vi "CRYGroup Manipulate.vi"(6 "sData In":string[](array[string]), 7 "sAction":string, 8 "sOption":string, 9 "nData":i32[](array[numeric]), 10 "Type":enum16{"Curves", "Values", "Results", "WFM"}(ring), 11 "Tree in":refnum<vi>) -> (0 "bData out":bool, 1 "sData Out":string[](array[string]), 2 "nData Out":i32[](array[numeric]), 3 "Tree Out":refnum<vi>)   [LabVIEW 2013]
uses:
  Global/CRYCurve Library Global.vi
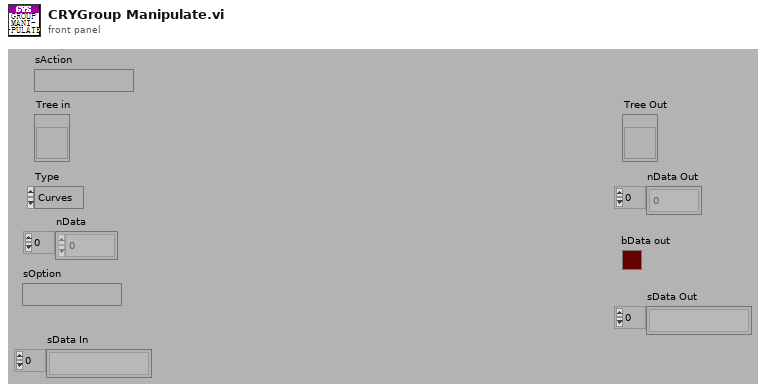
[diagram p1: front panel]
types:
  T1 = enum16{"OK", "Yes", "YesNo", "YesNoCancel", "ReplaceAppend"}
  T2 = typedef "CRYCurveLib Info Cluster.ctl" = cluster{"GroupingState":string}
  T3 = typedef "CRYStep.ctl" = cluster{"No.VI":i32, "Category":string, "StepName":string, "Seq setup flattened":string, "Comment":string, "Steps config.":bool[], "Jump config":i32[], "Start":dbl, "Increment":dbl, "Name":string, "Unit":string, "Y data":u16, "Y prefix":string, "Y dB ref":dbl, "Y unit":string, "Repeat State Array":cluster{"Start":dbl, "Increment":dbl, "Count":i32, "Num":i32}[]}
  T4 = cluster{"Tags":string[], "StepNo&Category":string}[]
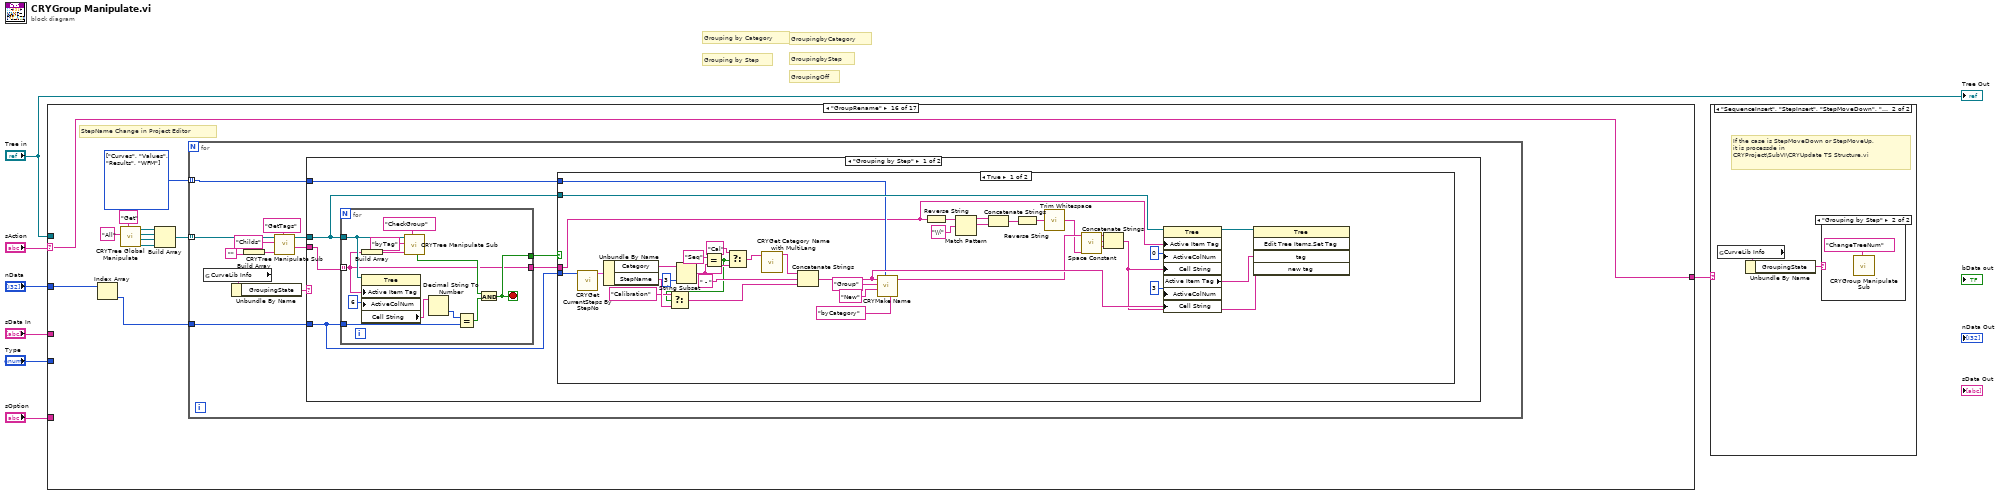
[diagram p0: block diagram]
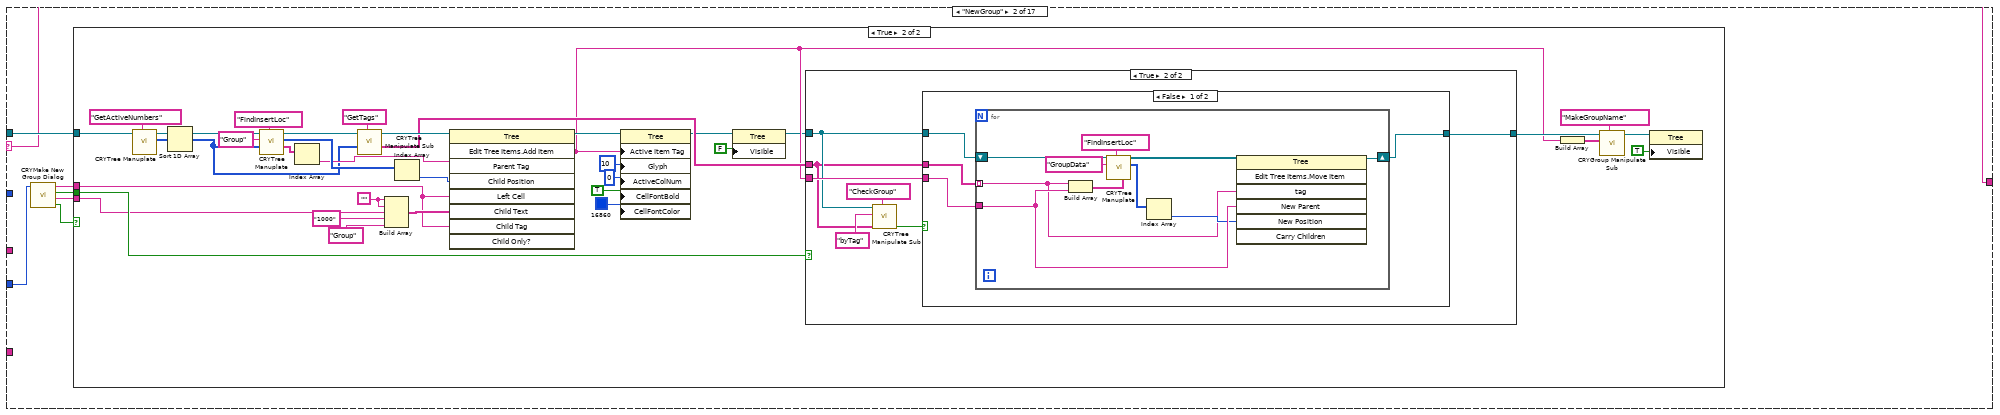
[diagram p5: hidden frame]
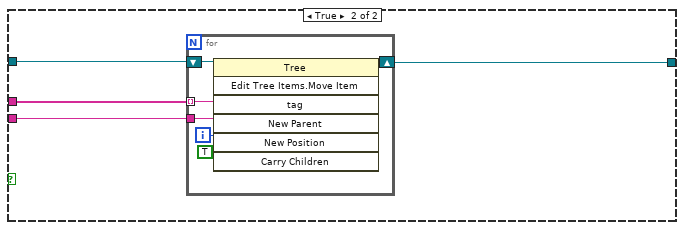
[diagram p8: hidden frame]
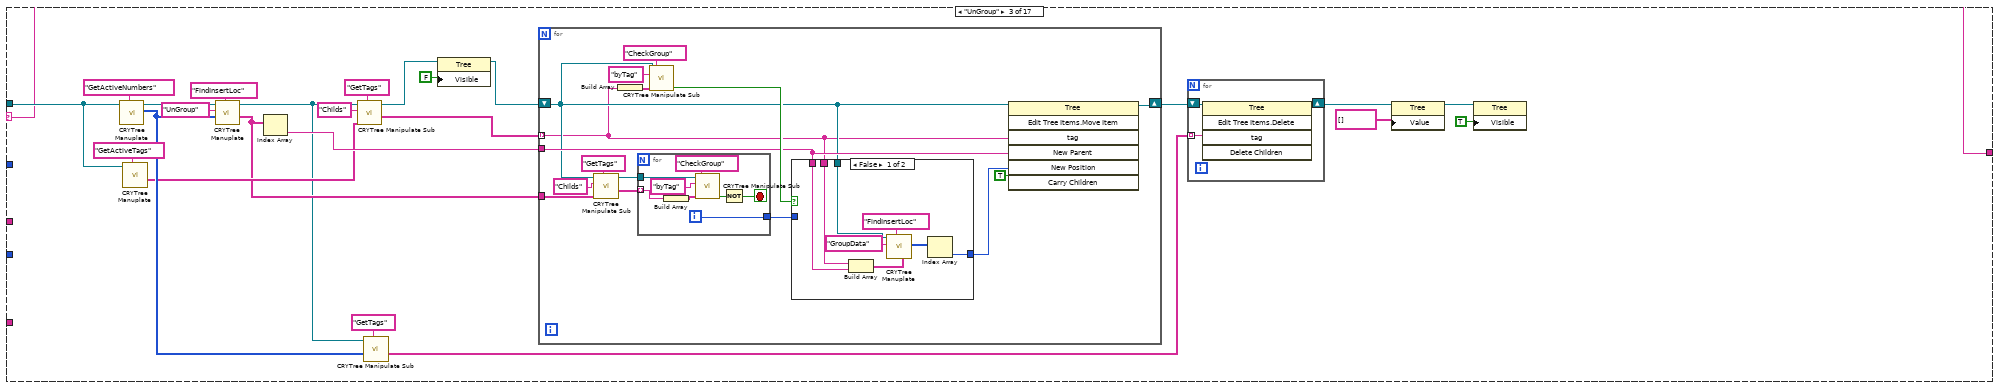
[diagram p9: hidden frame]
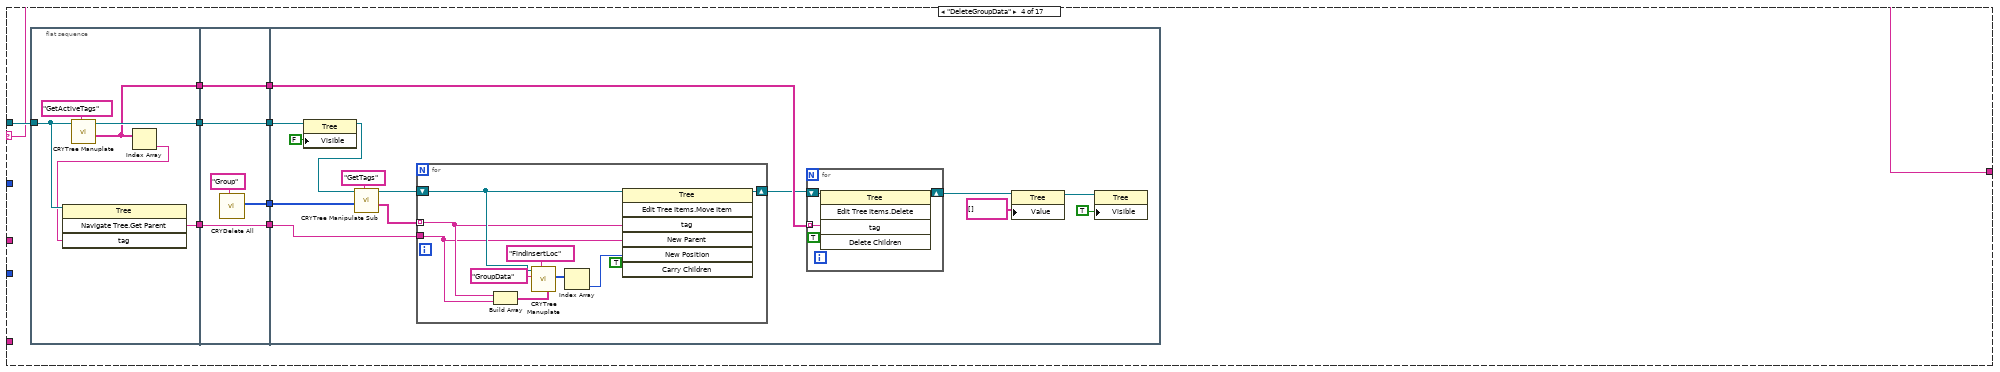
[diagram p11: hidden frame]
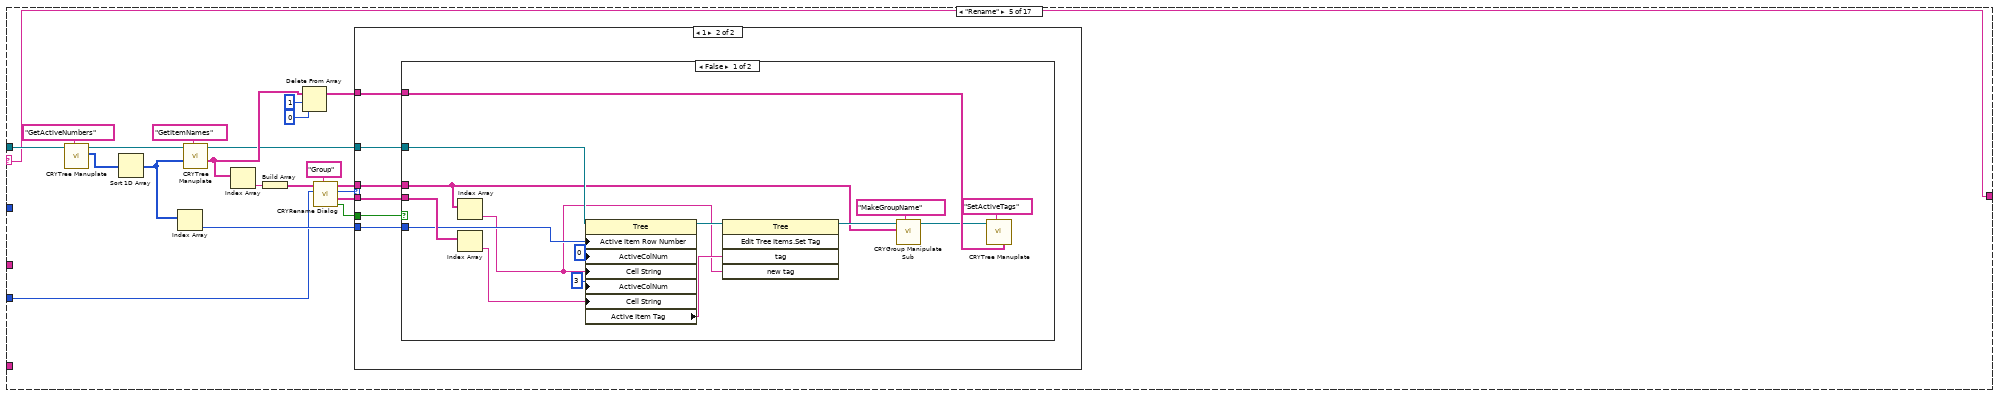
[diagram p12: hidden frame]
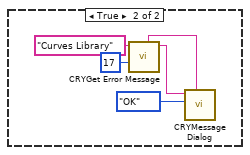
[diagram p14: hidden frame]
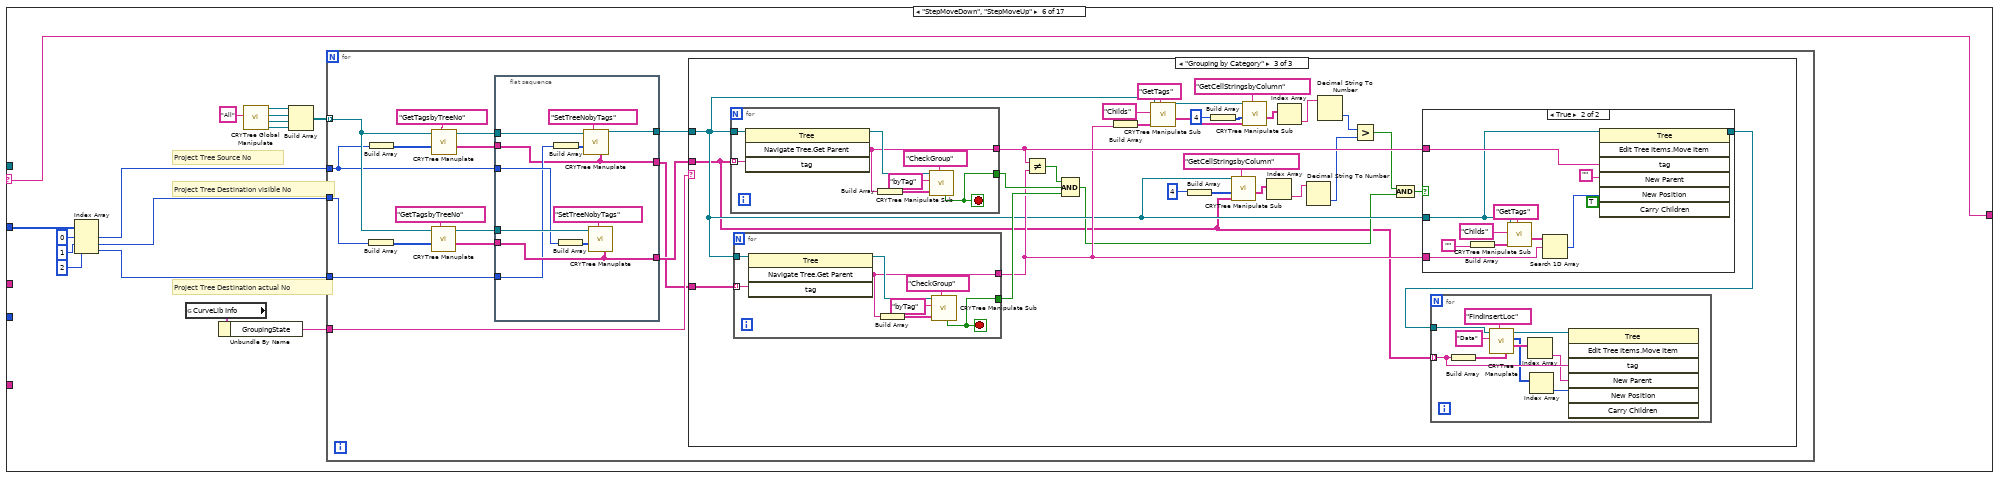
[diagram p15: hidden frame]
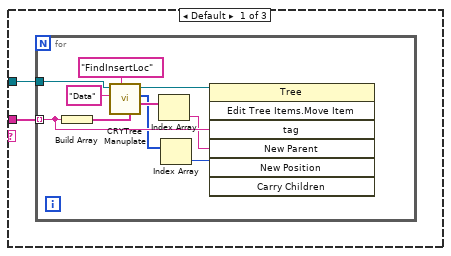
[diagram p16: hidden frame]
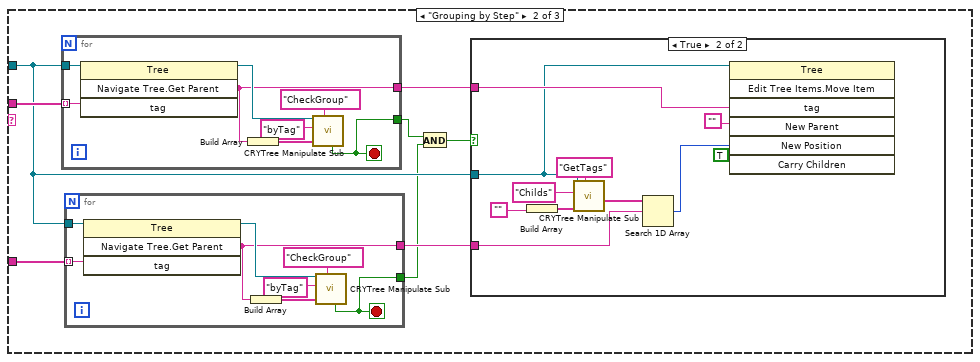
[diagram p17: hidden frame]
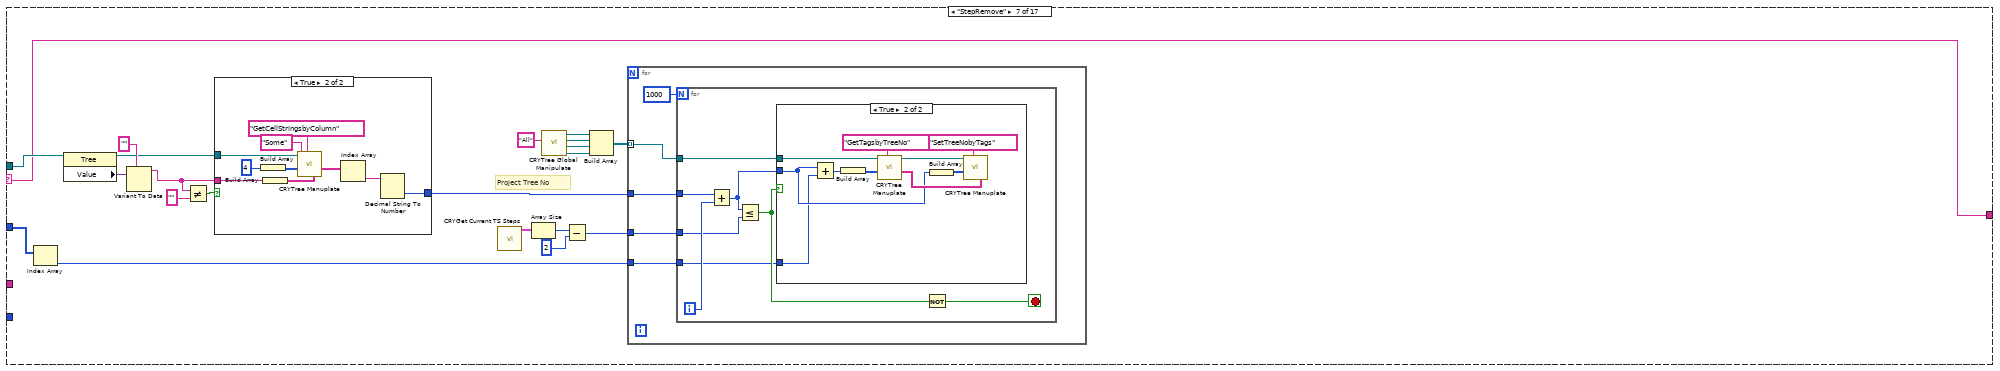
[diagram p20: hidden frame]
diagram:
  # "Grouping by Step"
  # "Grouping by Category"
  # "GroupingOff"
  # "GroupingbyStep"
  # "GroupingbyCategory"
  n1 = case shown="\"GroupRename\"" "sAction" {
    selector: "sAction" -> [w8 w9 w84 w145 w193 w242 w398 w452 w501 w555 w568 w581 w601 w709 w776 w835 w902]
    tunnel: "nData" -> [_ _ _ _ _ w247 w400 _ w503 w564 w569 w584 _ _ w790 w837 w916]
    tunnel: "Tree in" -> [_ w12 w88 w146 w202 _ w407 w459 w510 w562 w570 w585 _ _ w791 _ w937]
    tunnel: "Type" -> [_ w10 _ _ w194 _ _ _ _ _ _ _ _ _ _ _ w909]
    tunnel: "sOption" -> [_ _ _ _ _ _ _ _ _ _ _ _ _ w710 _ _ _]
    tunnel: [w8 w9 w84 w145 w193 w242 w398 w452 w501 w555 w568 w581 w601 w709 w776 w835 w902] -> w2
    tunnel: "sData In" -> [_ _ _ _ _ _ _ _ _ _ _ _ _ _ _ _ _]
    frame "None", Default {
    }
    frame "NewGroup" {
      n2 = call "CRYMake New Group Dialog.vi"("Type"=w10) -> ("Return Flag"=w14:bool, "Org Group Name"=w11:string, "InGroup?"=w13:bool, "New Group Name"=w15:string)  [unwired: 7 in]
      n3 = case shown="True" w14 {
        tunnel: w12 -> [_ w20]
        tunnel: w15 -> [_ w36]
        tunnel: w13 -> [_ w45]
        tunnel: w11 -> [_ w29]
        frame False {
        }
        frame True {
          w30 = ""
          n4 = call "CRYTree Manuplate.vi"("sAction"="GetActiveNumbers", "Tree in"=w20) -> ("nData Out"=w31:i32[], "Tree Out"=w46:refnum<vi>)  [unwired: 6 in, 2 out]
          n5 = Sort 1D Array(array=w31) -> (sorted array=w23:i32[])
          n6 = call "CRYTree Manuplate.vi"("sAction"="FindInsertLoc", "nData"=w23, "sOption"="Group" ("sData"), "Tree in"=w46) -> ("sData Out"=w39:string[], "nData Out"=w41:i32[], "Tree Out"=w37:refnum<vi>)  [unwired: 4 in, 1 out]
          n7 = Index Array(array=w39) -> (element=w35:string)  [unwired: 1 in]
          n8 = call "CRYTree Manipulate Sub.vi"("sAction"="GetTags", "nData"=w23, "Tree in"=w37) -> ("sData Out"=w42:string[], "Tree Out"=w43:refnum<vi>)  [unwired: 4 in, 3 out]
          n9 = Build Array(w30, w30, w29, "1000" ("element"), "Group" ("element")) -> (w49:string[])
          n10 = Index Array(array=w41) -> (element=w40:i32)  [unwired: 1 in]
          n11 = invoke class="Tree" method="Edit Tree Items.Add Item"(reference=w43, "Parent Tag"=w35, "Child Position"=w40, "Left Cell"=w36, "Child Text"=w49, "Child Tag"=w36) -> (reference out=w51:refnum<vi>, "Edit Tree Items:Add Item"=w26:string)  [unwired: 3 in, 7 out]
          n12 = property class="Tree"(reference=w51, "Active Item Tag"=w26, "Glyph"=10 ("Active Item:Symbol Index"), "ActiveColNum"=0 ("Active Cell:Active Column Number"), "CellFontBold"=TRUE ("Active Cell:Cell Font:Bold"), "CellFontColor"=u32 16860) -> (reference out=w18:refnum<vi>)  [unwired: 1 in, 1 out]
          n13 = property class="Tree"(reference=w18, "Visible"=FALSE) -> (reference out=w17:refnum<vi>)  [unwired: 1 in, 1 out]
          n14 = case shown="True" w45 {
            tunnel: w26 -> [_ w59]
            tunnel: w17 -> [w52 w55]
            tunnel: w42 -> [_ w54]
            tunnel: [w52 w58] -> w27
            frame False {
            }
            frame True {
              n15 = call "CRYTree Manipulate Sub.vi"("sAction"="CheckGroup", "sData"=w54, "sOption"="byTag", "Tree in"=w55) -> ("bData out"=w53:bool)  [unwired: 3 in, 4 out]
              n16 = case shown="False" w53 {
                tunnel: w59 -> [w61 w77]
                tunnel: [w60 w76] -> w58
                tunnel: w55 -> [w63 w75]
                tunnel: w54 -> [w62 w74]
                frame False {
                  n17 = for {
                    tunnel: w62 -> [w69] mode=indexing
                    tunnel: w61 -> [w72]
                    shift-right: [w71] -> w60
                    shift-left: w63 -> [w68]
                    n18 = Build Array(w69, w72) -> (w65:string[])
                    n19 = call "CRYTree Manuplate.vi"("sData"=w65, "sAction"="FindInsertLoc", "sOption"="GroupData", "Tree in"=w68) -> ("nData Out"=w64:i32[], "Tree Out"=w73:refnum<vi>)  [unwired: 4 in, 2 out]
                    n20 = Index Array(array=w64) -> (element=w70:i32)  [unwired: 1 in]
                    n21 = invoke class="Tree" method="Edit Tree Items.Move Item"(reference=w73, "tag"=w69, "New Parent"=w72, "New Position"=w70) -> (reference out=w71:refnum<vi>)  [unwired: 3 in, 6 out]
                  }
                }
                frame True {
                  n22 = for {
                    tunnel: w77 -> [w81]
                    tunnel: w74 -> [w82] mode=indexing
                    shift-right: [w78] -> w76
                    shift-left: w75 -> [w83]
                    i -> [w80]
                    n23 = invoke class="Tree" method="Edit Tree Items.Move Item"(reference=w83, "tag"=w82, "New Parent"=w81, "New Position"=w80, "Carry Children"=TRUE ("Carry Children?")) -> (reference out=w78:refnum<vi>)  [unwired: 2 in, 6 out]
                  }
                }
              }
            }
          }
          n24 = Build Array(w26) -> (w16:string[])
          n25 = call "CRYGroup Manipulate Sub.vi"("sAction"="MakeGroupName", "sData"=w16, "Tree in"=w27) -> ("Tree Out"=w21:refnum<vi>)  [unwired: 4 in, 4 out]
          n26 = property class="Tree"(reference=w21, "Visible"=TRUE) -> ()  [unwired: 1 in, 2 out]
        }
      }
    }
    frame "UnGroup" {
      n27 = call "CRYTree Manuplate.vi"("sAction"="GetActiveNumbers", "Tree in"=w88) -> ("nData Out"=w98:i32[], "Tree Out"=w106:refnum<vi>)  [unwired: 6 in, 2 out]
      n28 = call "CRYTree Manuplate.vi"("sAction"="GetActiveTags", "Tree in"=w88) -> ("sData Out"=w96:string[])  [unwired: 6 in, 3 out]
      n29 = call "CRYTree Manuplate.vi"("sAction"="FindInsertLoc", "nData"=w98, "sOption"="UnGroup" ("sData"), "Tree in"=w106) -> ("sData Out"=w95:string[], "Tree Out"=w92:refnum<vi>)  [unwired: 4 in, 2 out]
      n30 = Index Array(array=w95) -> (element=w102:string)  [unwired: 1 in]
      n31 = call "CRYTree Manipulate Sub.vi"("sAction"="GetTags", "sData"=w96, "sOption"="Childs" ("sData"), "Tree in"=w92) -> ("sData Out"=w103:string[], "Tree Out"=w86:refnum<vi>)  [unwired: 3 in, 3 out]
      n32 = call "CRYTree Manipulate Sub.vi"("sAction"="GetTags", "nData"=w98, "Tree in"=w92) -> ("sData Out"=w99:string[])  [unwired: 4 in, 4 out]
      n33 = property class="Tree"(reference=w86, "Visible"=FALSE) -> (reference out=w85:refnum<vi>)  [unwired: 1 in, 1 out]
      n34 = for {
        tunnel: w103 -> [w111] mode=indexing
        tunnel: w102 -> [w113]
        tunnel: w95 -> [w114]
        shift-right: [w124] -> w91
        shift-left: w85 -> [w112]
        n35 = call "CRYTree Manipulate Sub.vi"("sAction"="GetTags", "sData"=w114, "sOption"="Childs" ("sData"), "Tree in"=w112) -> ("sData Out"=w109:string[], "Tree Out"=w120:refnum<vi>)  [unwired: 3 in, 3 out]
        n36 = Build Array(w111) -> (w117:string[])
        n37 = for {
          tunnel: w109 -> [w138] mode=indexing
          tunnel: w120 -> [w140]
          tunnel: [w135] -> w115
          i -> [w135]
          stop <- w134 stop-if-true
          n38 = Build Array(w138) -> (w137:string[])
          n39 = call "CRYTree Manipulate Sub.vi"("sAction"="CheckGroup", "sData"=w137, "sOption"="byTag", "Tree in"=w140) -> ("bData out"=w136:bool)  [unwired: 3 in, 4 out]
          n40 = Not(x=w136) -> (.not. x?=w134:bool)
        }
        n41 = call "CRYTree Manipulate Sub.vi"("sAction"="CheckGroup", "sData"=w117, "sOption"="byTag", "Tree in"=w112) -> ("bData out"=w116:bool)  [unwired: 3 in, 4 out]
        n42 = case shown="False" w116 {
          tunnel: w115 -> [_ w133]
          tunnel: [w132 w133] -> w110
          tunnel: w113 -> [w131 _]
          tunnel: w112 -> [w130 _]
          tunnel: w111 -> [w129 _]
          frame False {
            n43 = Build Array(w129, w131) -> (w126:string[])
            n44 = call "CRYTree Manuplate.vi"("sData"=w126, "sAction"="FindInsertLoc", "sOption"="GroupData", "Tree in"=w130) -> ("nData Out"=w125:i32[])  [unwired: 4 in, 3 out]
            n45 = Index Array(array=w125) -> (element=w132:i32)  [unwired: 1 in]
          }
          frame True {
          }
        }
        n46 = invoke class="Tree" method="Edit Tree Items.Move Item"(reference=w112, "tag"=w111, "New Parent"=w113, "New Position"=w110, "Carry Children"=TRUE ("Carry Children?")) -> (reference out=w124:refnum<vi>)  [unwired: 2 in, 6 out]
      }
      n47 = for {
        tunnel: w99 -> [w143] mode=indexing
        shift-right: [w142] -> w94
        shift-left: w91 -> [w144]
        n48 = invoke class="Tree" method="Edit Tree Items.Delete"(reference=w144, "tag"=w143) -> (reference out=w142:refnum<vi>)  [unwired: 3 in, 4 out]
      }
      n49 = property class="Tree"(reference=w94, "Value"=string[] []) -> (reference out=w89:refnum<vi>)  [unwired: 1 in, 1 out]
      n50 = property class="Tree"(reference=w89, "Visible"=TRUE) -> ()  [unwired: 1 in, 2 out]
    }
    frame "DeleteGroupData" {
      n51 = flat-sequence {
        tunnel: w146 -> [w157]
        tunnel: [w158] -> w151
        tunnel: [w155] -> w149
        tunnel: [w154] -> w147
        tunnel: [w163] -> w153
        tunnel: [w162] -> w152
        tunnel: w151 -> [w163]
        tunnel: [w161] -> w150
        tunnel: w149 -> [w161]
        tunnel: [w160] -> w148
        tunnel: w147 -> [w160]
        tunnel: w153 -> [w166]
        tunnel: w152 -> [w170]
        tunnel: w150 -> [w173]
        tunnel: w148 -> [w172]
        frame #0 {
          n52 = call "CRYTree Manuplate.vi"("sAction"="GetActiveTags", "Tree in"=w157) -> ("sData Out"=w154:string[], "Tree Out"=w158:refnum<vi>)  [unwired: 6 in, 2 out]
          n53 = Index Array(array=w154) -> (element=w156:string)  [unwired: 1 in]
          n54 = invoke class="Tree" method="Navigate Tree.Get Parent"(reference=w157, "tag"=w156) -> ("Navigate Tree:Get Parent"=w155:string)  [unwired: 2 in, 3 out]
        }
        frame #1 {
          n55 = call "CRYDelete All.vi"("sAction"="Group") -> ("Deleted Rows"=w162:i32[])  [unwired: 9 in, 1 out]
        }
        frame #2 {
          n56 = property class="Tree"(reference=w166, "Visible"=FALSE) -> (reference out=w165:refnum<vi>)  [unwired: 1 in, 1 out]
          n57 = call "CRYTree Manipulate Sub.vi"("sAction"="GetTags", "nData"=w170, "Tree in"=w165) -> ("sData Out"=w175:string[], "Tree Out"=w174:refnum<vi>)  [unwired: 4 in, 3 out]
          n58 = for {
            tunnel: w173 -> [w180]
            tunnel: w175 -> [w181] mode=indexing
            shift-right: [w187] -> w171
            shift-left: w174 -> [w182]
            n59 = Build Array(w181, w180) -> (w185:string[])
            n60 = call "CRYTree Manuplate.vi"("sData"=w185, "sAction"="FindInsertLoc", "sOption"="GroupData", "Tree in"=w182) -> ("nData Out"=w186:i32[])  [unwired: 4 in, 3 out]
            n61 = Index Array(array=w186) -> (element=w179:i32)  [unwired: 1 in]
            n62 = invoke class="Tree" method="Edit Tree Items.Move Item"(reference=w182, "tag"=w181, "New Parent"=w180, "New Position"=w179, "Carry Children"=TRUE ("Carry Children?")) -> (reference out=w187:refnum<vi>)  [unwired: 2 in, 6 out]
          }
          n63 = for {
            tunnel: w172 -> [w191] mode=indexing
            shift-right: [w190] -> w178
            shift-left: w171 -> [w192]
            n64 = invoke class="Tree" method="Edit Tree Items.Delete"(reference=w192, "tag"=w191, "Delete Children"=TRUE ("Delete Children?")) -> (reference out=w190:refnum<vi>)  [unwired: 2 in, 4 out]
          }
          n65 = property class="Tree"(reference=w178, "Value"=string[] []) -> (reference out=w169:refnum<vi>)  [unwired: 1 in, 1 out]
          n66 = property class="Tree"(reference=w169, "Visible"=TRUE) -> ()  [unwired: 1 in, 2 out]
        }
      }
    }
    frame "Rename" {
      n67 = call "CRYTree Manuplate.vi"("sAction"="GetActiveNumbers", "Tree in"=w202) -> ("nData Out"=w201:i32[], "Tree Out"=w199:refnum<vi>)  [unwired: 6 in, 2 out]
      n68 = Sort 1D Array(array=w201) -> (sorted array=w196:i32[])
      n69 = Index Array(array=w196) -> (element=w195:i32)  [unwired: 1 in]
      n70 = call "CRYTree Manuplate.vi"("sAction"="GetItemNames", "nData"=w196, "Tree in"=w199) -> ("sData Out"=w198:string[], "Tree Out"=w197:refnum<vi>)  [unwired: 5 in, 2 out]
      n71 = Index Array(array=w198) -> (element=w210:string)  [unwired: 1 in]
      n72 = Build Array(w210) -> (w209:string[])
      n73 = Delete From Array(array=w198, length=1, index=0) -> (array with subset deleted=w204:string[])  [unwired: 1 out]
      n74 = call "CRYRename Dialog.vi"("sAction"="Group", "Type"=w194, "Name In"=w209) -> ("bReturn"=w207:bool, "Org Name"=w208:string[], "Index"=w213:i32, "New Name"=w212:string[])  [unwired: 1 in, 3 out]
      n75 = case shown="1" w213 {
        tunnel: w212 -> [_ w218]
        tunnel: w197 -> [_ w219]
        tunnel: w208 -> [_ w217]
        tunnel: w207 -> [_ w216]
        tunnel: w204 -> [_ w215]
        tunnel: w195 -> [_ w214]
        frame 0, Default {
        }
        frame 1 {
          n76 = case shown="False" w216 {
            tunnel: w219 -> [w225 _]
            tunnel: w218 -> [w220 _]
            tunnel: w217 -> [w232 _]
            tunnel: w215 -> [w227 _]
            tunnel: w214 -> [w226 _]
            frame False {
              n77 = Index Array(array=w220) -> (element=w222:string)  [unwired: 1 in]
              n78 = Index Array(array=w232) -> (element=w230:string)  [unwired: 1 in]
              n79 = property class="Tree"(reference=w225, "Active Item Row Number"=w226, "ActiveColNum"=0 ("Active Cell:Active Column Number"), "Cell String"=w222, "ActiveColNum"=3 ("Active Cell:Active Column Number"), "Cell String"=w230) -> (reference out=w233:refnum<vi>, "Active Item Tag"=w229:string)  [unwired: 1 in, 1 out]
              n80 = invoke class="Tree" method="Edit Tree Items.Set Tag"(reference=w233, "tag"=w229, "new tag"=w222) -> (reference out=w223:refnum<vi>)  [unwired: 2 in, 4 out]
              n81 = call "CRYGroup Manipulate Sub.vi"("sAction"="MakeGroupName", "sData"=w220, "Tree in"=w223) -> ("Tree Out"=w221:refnum<vi>)  [unwired: 4 in, 4 out]
              n82 = call "CRYTree Manuplate.vi"("sData"=w227, "sAction"="SetActiveTags", "Tree in"=w221) -> ()  [unwired: 5 in, 4 out]
            }
            frame True {
              n83 = call "CRYGet Error Message.vi"("Error No"=17, "Kind"="Curves Library") -> ("Message"=w236:string, "Window Title"=w235:string)  [unwired: 4 in, 4 out]
              n84 = call "CRYMessage Dialog.vi"("Window Title"=w235, "YesNoCancel"=T1."OK", "Message Content"=w236) -> ()  [unwired: 7 in, 2 out]
            }
          }
        }
      }
    }
    frame "StepMoveDown", "StepMoveUp" {
      # "Project Tree Destination actual No"
      # "Project Tree Destination visible No"
      # "Project Tree Source No"
      n85 = Index Array(array=w247, index #1=0 ("index"), index #2=1 ("index"), index #3=2 ("index")) -> (element #1=w249:i32, element #2=w248:i32, element #3=w246:i32)
      n86 = global read "CRYCurve Library Global.vi" "CurveLib Info"() -> (w241:T2)
      n87 = Unbundle By Name(w241) -> ("GroupingState"=w240:string)
      n88 = call "CRYTree Global Manipulate.vi"("sOption"="All") -> ("WFM Tree"=w251:refnum<vi>, "Results Tree"=w252:refnum<vi>, "Values Tree"=w253:refnum<vi>, "Tree/Curve Tree"=w254:refnum<vi>)  [unwired: 7 in]
      n89 = Build Array(w254, w253, w252, w251) -> (w250:refnum<vi>[])
      n90 = for {
        tunnel: w250 -> [w267] mode=indexing
        tunnel: w249 -> [w260]
        tunnel: w248 -> [w265]
        tunnel: w246 -> [w259]
        tunnel: w240 -> [w257]
        n91 = Build Array(w265) -> (w269:i32[])
        n92 = Build Array(w260) -> (w270:i32[])
        n93 = call "CRYTree Manuplate.vi"("sAction"="GetTagsbyTreeNo", "nData"=w269, "Tree in"=w267) -> ("sData Out"=w262:string[], "Tree Out"=w264:refnum<vi>)  [unwired: 5 in, 2 out]
        n94 = call "CRYTree Manuplate.vi"("sAction"="GetTagsbyTreeNo", "nData"=w270, "Tree in"=w267) -> ("sData Out"=w263:string[], "Tree Out"=w266:refnum<vi>)  [unwired: 5 in, 2 out]
        n95 = flat-sequence {
          tunnel: w266 -> [w396]
          tunnel: w264 -> [w392]
          tunnel: [w391] -> w258
          tunnel: w263 -> [w387]
          tunnel: w262 -> [w390]
          tunnel: [w390] -> w261
          tunnel: w260 -> [w389]
          tunnel: w259 -> [w388]
          tunnel: [w387] -> w256
          frame #0 {
            n96 = Build Array(w388) -> (w395:i32[])
            n97 = Build Array(w389) -> (w394:i32[])
            n98 = call "CRYTree Manuplate.vi"("sData"=w387, "sAction"="SetTreeNobyTags", "nData"=w395, "Tree in"=w396) -> ("Tree Out"=w391:refnum<vi>)  [unwired: 4 in, 3 out]
            n99 = call "CRYTree Manuplate.vi"("sData"=w390, "sAction"="SetTreeNobyTags", "nData"=w394, "Tree in"=w392) -> ()  [unwired: 4 in, 4 out]
          }
        }
        n100 = case shown="\"Grouping by Category\"" w257 {
          tunnel: w261 -> [w273 w291 w319]
          tunnel: w258 -> [w272 w287 w331]
          tunnel: w256 -> [_ w289 w345]
          frame Default {
            n101 = for {
              tunnel: w273 -> [w279] mode=indexing
              tunnel: w272 -> [w274]
              n102 = Build Array(w279) -> (w281:string[])
              n103 = call "CRYTree Manuplate.vi"("sData"=w281, "sAction"="FindInsertLoc", "sOption"="Data", "Tree in"=w274) -> ("sData Out"=w278:string[], "nData Out"=w276:i32[], "Tree Out"=w280:refnum<vi>)  [unwired: 4 in, 1 out]
              n104 = Index Array(array=w278) -> (element=w277:string)  [unwired: 1 in]
              n105 = Index Array(array=w276) -> (element=w275:i32)  [unwired: 1 in]
              n106 = invoke class="Tree" method="Edit Tree Items.Move Item"(reference=w280, "tag"=w279, "New Parent"=w277, "New Position"=w275) -> ()  [unwired: 3 in, 7 out]
            }
          }
          frame "Grouping by Step" {
            n107 = for {
              tunnel: w291 -> [w313] mode=indexing
              tunnel: [w312] -> w290
              tunnel: w287 -> [w318]
              tunnel: [w311] -> w286
              stop <- w311 stop-if-true
              n108 = invoke class="Tree" method="Navigate Tree.Get Parent"(reference=w318, "tag"=w313) -> (reference out=w314:refnum<vi>, "Navigate Tree:Get Parent"=w312:string)  [unwired: 2 in, 2 out]
              n109 = Build Array(w312) -> (w315:string[])
              n110 = call "CRYTree Manipulate Sub.vi"("sAction"="CheckGroup", "sData"=w315, "sOption"="byTag", "Tree in"=w314) -> ("bCategory"=w311:bool)  [unwired: 3 in, 4 out]
            }
            n111 = for {
              tunnel: w289 -> [w305] mode=indexing
              tunnel: [w304] -> w288
              tunnel: w287 -> [w310]
              tunnel: [w303] -> w285
              stop <- w303 stop-if-true
              n112 = invoke class="Tree" method="Navigate Tree.Get Parent"(reference=w310, "tag"=w305) -> (reference out=w306:refnum<vi>, "Navigate Tree:Get Parent"=w304:string)  [unwired: 2 in, 2 out]
              n113 = Build Array(w304) -> (w307:string[])
              n114 = call "CRYTree Manipulate Sub.vi"("sAction"="CheckGroup", "sData"=w307, "sOption"="byTag", "Tree in"=w306) -> ("bCategory"=w303:bool)  [unwired: 3 in, 4 out]
            }
            n115 = And(x=w286, y=w285) -> (x .and. y?=w284:bool)
            n116 = case shown="True" w284 {
              tunnel: w290 -> [_ w295]
              tunnel: w288 -> [_ w293]
              tunnel: w287 -> [_ w292]
              frame False {
              }
              frame True {
                n117 = Build Array("") -> (w299:string[])
                n118 = call "CRYTree Manipulate Sub.vi"("sAction"="GetTags", "sData"=w299, "sOption"="Childs", "Tree in"=w292) -> ("sData Out"=w296:string[])  [unwired: 3 in, 4 out]
                n119 = Search 1D Array(1D array=w296, element=w293) -> (index of element=w294:i32)  [unwired: 1 in]
                n120 = invoke class="Tree" method="Edit Tree Items.Move Item"(reference=w292, "tag"=w295, "New Parent"="", "New Position"=w294, "Carry Children"=TRUE ("Carry Children?")) -> ()  [unwired: 2 in, 7 out]
              }
            }
          }
          frame "Grouping by Category" {
            n121 = for {
              tunnel: w319 -> [w381] mode=indexing
              tunnel: [w380] -> w344
              tunnel: w331 -> [w386]
              tunnel: [w379] -> w347
              stop <- w379 stop-if-true
              n122 = invoke class="Tree" method="Navigate Tree.Get Parent"(reference=w386, "tag"=w381) -> (reference out=w382:refnum<vi>, "Navigate Tree:Get Parent"=w380:string)  [unwired: 2 in, 2 out]
              n123 = Build Array(w380) -> (w383:string[])
              n124 = call "CRYTree Manipulate Sub.vi"("sAction"="CheckGroup", "sData"=w383, "sOption"="byTag", "Tree in"=w382) -> ("bCategory"=w379:bool)  [unwired: 3 in, 4 out]
            }
            n125 = for {
              tunnel: w345 -> [w373] mode=indexing
              tunnel: [w372] -> w339
              tunnel: w331 -> [w378]
              tunnel: [w371] -> w346
              stop <- w371 stop-if-true
              n126 = invoke class="Tree" method="Navigate Tree.Get Parent"(reference=w378, "tag"=w373) -> (reference out=w374:refnum<vi>, "Navigate Tree:Get Parent"=w372:string)  [unwired: 2 in, 2 out]
              n127 = Build Array(w372) -> (w375:string[])
              n128 = call "CRYTree Manipulate Sub.vi"("sAction"="CheckGroup", "sData"=w375, "sOption"="byTag", "Tree in"=w374) -> ("bCategory"=w371:bool)  [unwired: 3 in, 4 out]
            }
            n129 = Not Equal?(x=w344, y=w339) -> (x != y?=w343:bool)
            n130 = Compound Arithmetic op=AND(w343, w347, w346) -> (w329:bool)
            n131 = Build Array(w339) -> (w341:string[])
            n132 = call "CRYTree Manipulate Sub.vi"("sAction"="GetTags", "sData"=w341, "sOption"="Childs", "Tree in"=w331) -> ("sData Out"=w336:string[], "Tree Out"=w337:refnum<vi>)  [unwired: 3 in, 3 out]
            n133 = Build Array(4 ("nData 2")) -> (w333:i32[])
            n134 = Build Array(4 ("nData 2")) -> (w334:i32[])
            n135 = call "CRYTree Manipulate Sub.vi"("sAction"="GetCellStringsbyColumn", "sData"=w319, "nData"=w333, "Tree in"=w331) -> ("sData Out"=w323:string[])  [unwired: 3 in, 4 out]
            n136 = call "CRYTree Manipulate Sub.vi"("sAction"="GetCellStringsbyColumn", "sData"=w336, "nData"=w334, "Tree in"=w337) -> ("sData Out"=w326:string[])  [unwired: 3 in, 4 out]
            n137 = Index Array(array=w323) -> (element=w322:string)  [unwired: 1 in]
            n138 = Index Array(array=w326) -> (element=w325:string)  [unwired: 1 in]
            n139 = Decimal String To Number(string=w322) -> (number=w321:i32)  [unwired: 2 in, 1 out]
            n140 = Decimal String To Number(string=w325) -> (number=w324:i32)  [unwired: 2 in, 1 out]
            n141 = Greater?(x=w324, y=w321) -> (0:w328:bool)
            n142 = Compound Arithmetic op=AND(w328, w329) -> (w327:bool)
            n143 = case shown="True" w327 {
              tunnel: w344 -> [_ w363]
              tunnel: w339 -> [_ w361]
              tunnel: w331 -> [w358 w360]
              tunnel: [w358 w359] -> w320
              frame False {
              }
              frame True {
                n144 = Build Array("") -> (w367:string[])
                n145 = call "CRYTree Manipulate Sub.vi"("sAction"="GetTags", "sData"=w367, "sOption"="Childs", "Tree in"=w360) -> ("sData Out"=w364:string[])  [unwired: 3 in, 4 out]
                n146 = Search 1D Array(1D array=w364, element=w361) -> (index of element=w362:i32)  [unwired: 1 in]
                n147 = invoke class="Tree" method="Edit Tree Items.Move Item"(reference=w360, "tag"=w363, "New Parent"="", "New Position"=w362, "Carry Children"=TRUE ("Carry Children?")) -> (reference out=w359:refnum<vi>)  [unwired: 2 in, 6 out]
              }
            }
            n148 = for {
              tunnel: w319 -> [w353] mode=indexing
              tunnel: w320 -> [w348]
              n149 = Build Array(w353) -> (w355:string[])
              n150 = call "CRYTree Manuplate.vi"("sData"=w355, "sAction"="FindInsertLoc", "sOption"="Data", "Tree in"=w348) -> ("sData Out"=w352:string[], "nData Out"=w350:i32[], "Tree Out"=w354:refnum<vi>)  [unwired: 4 in, 1 out]
              n151 = Index Array(array=w352) -> (element=w351:string)  [unwired: 1 in]
              n152 = Index Array(array=w350) -> (element=w349:i32)  [unwired: 1 in]
              n153 = invoke class="Tree" method="Edit Tree Items.Move Item"(reference=w354, "tag"=w353, "New Parent"=w351, "New Position"=w349) -> ()  [unwired: 3 in, 7 out]
            }
          }
        }
      }
    }
    frame "StepRemove" {
      # "Project Tree No"
      n154 = Index Array(array=w400) -> (element=w399:i32)  [unwired: 1 in]
      n155 = property class="Tree"(reference=w407) -> (reference out=w406:refnum<vi>, "Value"=w409:variant)  [unwired: 1 in, 1 out]
      n156 = Variant To Data(type="" ("y"), Variant=w409) -> (data=w405:string)  [unwired: 1 in, 1 out]
      n157 = Not Equal?(x=w405, y="") -> (x != y?=w417:bool)
      n158 = case shown="True" w417 {
        tunnel: [_ w451] -> w410
        tunnel: w406 -> [_ w442]
        tunnel: w405 -> [_ w443]
        frame False {
        }
        frame True {
          n159 = Build Array(4 ("nData 2")) -> (w449:i32[])
          n160 = Build Array(w443) -> (w446:string[])
          n161 = call "CRYTree Manuplate.vi"("sData"=w446, "sAction"="GetCellStringsbyColumn", "nData"=w449, "sOption"="Some", "Tree in"=w442) -> ("sData Out"=w445:string[])  [unwired: 3 in, 3 out]
          n162 = Index Array(array=w445) -> (element=w444:string)  [unwired: 1 in]
          n163 = Decimal String To Number(string=w444) -> (number=w451:i32)  [unwired: 2 in, 1 out]
        }
      }
      n164 = call "CRYGet Current TS Steps.vi"() -> ("Steps"=w404:T3[])  [unwired: 7 in, 4 out]
      n165 = Array Size(array=w404) -> (size(s)=w403:i32)
      n166 = call "CRYTree Global Manipulate.vi"("sOption"="All") -> ("WFM Tree"=w412:refnum<vi>, "Results Tree"=w413:refnum<vi>, "Values Tree"=w414:refnum<vi>, "Tree/Curve Tree"=w415:refnum<vi>)  [unwired: 7 in]
      n167 = Subtract(x=w403, y=2) -> (x-y=w402:i32)
      n168 = Build Array(w415, w414, w413, w412) -> (w411:refnum<vi>[])
      n169 = for {
        tunnel: w411 -> [w423] mode=indexing
        tunnel: w410 -> [w422]
        tunnel: w402 -> [w421]
        tunnel: w399 -> [w419]
        n170 = for {
          N: 1000 -> [_]
          tunnel: w423 -> [w431]
          tunnel: w422 -> [w429]
          tunnel: w421 -> [w428]
          tunnel: w419 -> [w424]
          i -> [w430]
          stop <- w426 stop-if-true
          n171 = Add(x=w429, y=w430) -> (x+y=w425:i32)
          n172 = Less Or Equal?(x=w425, y=w428) -> (x <= y?=w427:bool)
          n173 = case shown="True" w427 {
            tunnel: w431 -> [_ w439]
            tunnel: w425 -> [_ w434]
            tunnel: w424 -> [_ w433]
            frame False {
            }
            frame True {
              n174 = Add(x=w434, y=w433) -> (x+y=w432:i32)
              n175 = Build Array(w432) -> (w440:i32[])
              n176 = call "CRYTree Manuplate.vi"("sAction"="GetTagsbyTreeNo", "nData"=w440, "Tree in"=w439) -> ("sData Out"=w436:string[], "Tree Out"=w437:refnum<vi>)  [unwired: 5 in, 2 out]
              n177 = Build Array(w434) -> (w435:i32[])
              n178 = call "CRYTree Manuplate.vi"("sData"=w436, "sAction"="SetTreeNobyTags", "nData"=w435, "Tree in"=w437) -> ()  [unwired: 4 in, 4 out]
            }
          }
          n179 = Not(x=w427) -> (.not. x?=w426:bool)
        }
      }
    }
    frame "StepInsert" {
      # "Project Tree No"
      n180 = property class="Tree"(reference=w459) -> (reference out=w458:refnum<vi>, "Value"=w461:variant)  [unwired: 1 in, 1 out]
      n181 = Variant To Data(type="" ("y"), Variant=w461) -> (data=w457:string)  [unwired: 1 in, 1 out]
      n182 = Not Equal?(x=w457, y="") -> (x != y?=w469:bool)
      n183 = case shown="True" w469 {
        tunnel: [_ w500] -> w462
        tunnel: w458 -> [_ w491]
        tunnel: w457 -> [_ w492]
        frame False {
        }
        frame True {
          n184 = Build Array(4 ("nData 2")) -> (w498:i32[])
          n185 = Build Array(w492) -> (w495:string[])
          n186 = call "CRYTree Manuplate.vi"("sData"=w495, "sAction"="GetCellStringsbyColumn", "nData"=w498, "sOption"="Some", "Tree in"=w491) -> ("sData Out"=w494:string[])  [unwired: 3 in, 3 out]
          n187 = Index Array(array=w494) -> (element=w493:string)  [unwired: 1 in]
          n188 = Decimal String To Number(string=w493) -> (number=w500:i32)  [unwired: 2 in, 1 out]
        }
      }
      n189 = call "CRYGet Current TS Steps.vi"() -> ("Steps"=w456:T3[])  [unwired: 7 in, 4 out]
      n190 = Array Size(array=w456) -> (size(s)=w455:i32)
      n191 = call "CRYTree Global Manipulate.vi"("sOption"="All") -> ("WFM Tree"=w464:refnum<vi>, "Results Tree"=w465:refnum<vi>, "Values Tree"=w466:refnum<vi>, "Tree/Curve Tree"=w467:refnum<vi>)  [unwired: 7 in]
      n192 = Subtract(x=w455, y=3) -> (x-y=w454:i32)
      n193 = Build Array(w467, w466, w465, w464) -> (w463:refnum<vi>[])
      n194 = for {
        tunnel: w463 -> [w474] mode=indexing
        tunnel: w462 -> [w473]
        tunnel: w454 -> [w472]
        n195 = for {
          N: 1000 -> [_]
          tunnel: w474 -> [w481]
          tunnel: w473 -> [w475]
          tunnel: w472 -> [w478]
          i -> [w477]
          stop <- w479 stop-if-true
          n196 = Subtract(x=w478, y=w477) -> (x-y=w476:i32)
          n197 = Greater Or Equal?(x=w476, y=w475) -> (x >= y?=w480:bool)
          n198 = case shown="True" w480 {
            tunnel: w481 -> [_ w488]
            tunnel: w476 -> [_ w482]
            frame False {
            }
            frame True {
              n199 = Increment(x=w482) -> (x+1=w483:i32)
              n200 = Build Array(w482) -> (w489:i32[])
              n201 = call "CRYTree Manuplate.vi"("sAction"="GetTagsbyTreeNo", "nData"=w489, "Tree in"=w488) -> ("sData Out"=w485:string[], "Tree Out"=w486:refnum<vi>)  [unwired: 5 in, 2 out]
              n202 = Build Array(w483) -> (w484:i32[])
              n203 = call "CRYTree Manuplate.vi"("sData"=w485, "sAction"="SetTreeNobyTags", "nData"=w484, "Tree in"=w486) -> ()  [unwired: 4 in, 4 out]
            }
          }
          n204 = Not(x=w480) -> (.not. x?=w479:bool)
        }
      }
    }
    frame "SequenceInsert" {
      # "Project Tree No"
      n205 = Index Array(array=w503) -> (element=w502:i32)  [unwired: 1 in]
      n206 = property class="Tree"(reference=w510) -> (reference out=w509:refnum<vi>, "Value"=w512:variant)  [unwired: 1 in, 1 out]
      n207 = Variant To Data(type="" ("y"), Variant=w512) -> (data=w508:string)  [unwired: 1 in, 1 out]
      n208 = Not Equal?(x=w508, y="") -> (x != y?=w520:bool)
      n209 = case shown="True" w520 {
        tunnel: [_ w554] -> w513
        tunnel: w509 -> [_ w545]
        tunnel: w508 -> [_ w546]
        frame False {
        }
        frame True {
          n210 = Build Array(4 ("nData 2")) -> (w552:i32[])
          n211 = Build Array(w546) -> (w549:string[])
          n212 = call "CRYTree Manuplate.vi"("sData"=w549, "sAction"="GetCellStringsbyColumn", "nData"=w552, "sOption"="Some", "Tree in"=w545) -> ("sData Out"=w548:string[])  [unwired: 3 in, 3 out]
          n213 = Index Array(array=w548) -> (element=w547:string)  [unwired: 1 in]
          n214 = Decimal String To Number(string=w547) -> (number=w554:i32)  [unwired: 2 in, 1 out]
        }
      }
      n215 = call "CRYGet Current TS Steps.vi"() -> ("Steps"=w507:T3[])  [unwired: 7 in, 4 out]
      n216 = Array Size(array=w507) -> (size(s)=w506:i32)
      n217 = call "CRYTree Global Manipulate.vi"("sOption"="All") -> ("WFM Tree"=w515:refnum<vi>, "Results Tree"=w516:refnum<vi>, "Values Tree"=w517:refnum<vi>, "Tree/Curve Tree"=w518:refnum<vi>)  [unwired: 7 in]
      n218 = Subtract(x=w506, y=3) -> (x-y=w505:i32)
      n219 = Build Array(w518, w517, w516, w515) -> (w514:refnum<vi>[])
      n220 = for {
        tunnel: w514 -> [w526] mode=indexing
        tunnel: w513 -> [w525]
        tunnel: w505 -> [w524]
        tunnel: w502 -> [w522]
        n221 = for {
          N: 1000 -> [_]
          tunnel: w526 -> [w534]
          tunnel: w525 -> [w528]
          tunnel: w524 -> [w531]
          tunnel: w522 -> [w527]
          i -> [w530]
          stop <- w532 stop-if-true
          n222 = Subtract(x=w531, y=w530) -> (x-y=w529:i32)
          n223 = Greater Or Equal?(x=w529, y=w528) -> (x >= y?=w533:bool)
          n224 = case shown="True" w533 {
            tunnel: w534 -> [_ w542]
            tunnel: w529 -> [_ w537]
            tunnel: w527 -> [_ w536]
            frame False {
            }
            frame True {
              n225 = Add(x=w537, y=w536) -> (x+y=w535:i32)
              n226 = Build Array(w537) -> (w543:i32[])
              n227 = call "CRYTree Manuplate.vi"("sAction"="GetTagsbyTreeNo", "nData"=w543, "Tree in"=w542) -> ("sData Out"=w539:string[], "Tree Out"=w540:refnum<vi>)  [unwired: 5 in, 2 out]
              n228 = Build Array(w535) -> (w538:i32[])
              n229 = call "CRYTree Manuplate.vi"("sData"=w539, "sAction"="SetTreeNobyTags", "nData"=w538, "Tree in"=w540) -> ()  [unwired: 4 in, 4 out]
            }
          }
          n230 = Not(x=w533) -> (.not. x?=w532:bool)
        }
      }
    }
    frame "DeletebyStepNo" {
      n231 = Index Array(array=w564) -> (element=w563:i32)  [unwired: 1 in]
      n232 = call "CRYGet Tree Number by StepNo.vi"("sOption"="ActualNumber", "Step Setup VI No"=w563) -> ("Number in Tree"=w560:i32)  [unwired: 8 in, 1 out]
      n233 = Build Array(w560) -> (w559:i32[])
      n234 = call "CRYTree Manuplate.vi"("sAction"="GetTagsbyTreeNo", "nData"=w559, "Tree in"=w562) -> ("sData Out"=w557:string[], "Tree Out"=w558:refnum<vi>)  [unwired: 5 in, 2 out]
      n235 = for {
        shift-right: [w567] -> _
        shift-left: w558 -> [w566]
        tunnel: w557 -> [w565] mode=indexing
        n236 = invoke class="Tree" method="Edit Tree Items.Delete"(reference=w566, "tag"=w565) -> (reference out=w567:refnum<vi>)  [unwired: 3 in, 4 out]
      }
    }
    frame "GetGroupData" {
      n237 = call "CRYTree Manipulate Sub.vi"("sAction"="CheckGroup", "nData"=w569, "sOption"="byNum", "Tree in"=w570) -> ("bData out"=w572:bool, "Tree Out"=w573:refnum<vi>)  [unwired: 3 in, 3 out]
      n238 = case shown="True" w572 {
        tunnel: w573 -> [_ w580]
        tunnel: w569 -> [w576 w578]
        tunnel: [w576 w577] -> w571
        frame False {
        }
        frame True {
          n239 = call "CRYTree Manuplate.vi"("sAction"="GetAllChild", "nData"=w578, "Tree in"=w580) -> ("nData Out"=w577:i32[])  [unwired: 5 in, 3 out]
        }
      }
      n240 = local write "nData Out"(w571) -> ()
    }
    frame "GetDragData" {
      n241 = for {
        tunnel: w585 -> [w591]
        tunnel: w584 -> [w590] mode=indexing
        shift-right: [w586] -> w582
        shift-left: i32[] [] ("nData") -> [w588]
        n242 = Build Array(w590) -> (w589:i32[])
        n243 = call "CRYTree Manipulate Sub.vi"("sAction"="CheckGroup", "nData"=w589, "sOption"="byNum", "Tree in"=w591) -> ("bData out"=w592:bool, "Tree Out"=w593:refnum<vi>)  [unwired: 3 in, 3 out]
        n244 = case shown="True" w592 {
          tunnel: w593 -> [_ w600]
          tunnel: w589 -> [w596 w598]
          tunnel: [w596 w597] -> w587
          frame False {
          }
          frame True {
            n245 = call "CRYTree Manuplate.vi"("sAction"="GetAllChild", "nData"=w598, "Tree in"=w600) -> ("nData Out"=w597:i32[])  [unwired: 5 in, 3 out]
          }
        }
        n246 = Insert Into Array(array=w588, new element=w587) -> (w586:i32[])  [unwired: 1 in]
      }
      n247 = local write "nData Out"(w582) -> ()
    }
    frame "GroupingbyCategory", "GroupingbyStep" {
      w602 = enum16{"Curves", "Values", "Results", "WFM"}[] [enum."Curves", enum."Values", enum."Results", enum."WFM"] items=["Curves", "Values", "Results", "WFM"]
      n248 = for {
        tunnel: w602 -> [w605] mode=indexing
        tunnel: w601 -> [w603]
        n249 = call "CRYTree Global Manipulate.vi"("sAction"="Get", "Type In"=w605) -> ("Tree/Curve Tree"=w609:refnum<vi>)  [unwired: 6 in, 3 out]
        n250 = call "CRYTree Manuplate.vi"("sAction"="FindInsertLoc", "sOption"="Grouping" ("sData"), "Tree in"=w609) -> ("bResult Out"=w608:bool, "sData Out"=w607:string[], "nData Out"=w604:i32[], "Tree Out"=w606:refnum<vi>)  [unwired: 5 in]
        n251 = case shown="True" w608 {
          tunnel: w607 -> [_ w627]
          tunnel: w606 -> [w613 w621]
          tunnel: w605 -> [_ w615]
          tunnel: w604 -> [_ w628]
          tunnel: w603 -> [_ w616]
          frame False {
            n252 = property class="Tree"(reference=w613, "Visible"=TRUE) -> ()  [unwired: 1 in, 2 out]
          }
          frame True {
            n253 = Index Array(array=w628) -> (element=w630:i32)  [unwired: 1 in]
            n254 = call "CRYGroup Manipulate Sub.vi"("Type"=w615, "sAction"=w616, "sData"=w627, "Tree in"=w621) -> ("Step&Tags Out"=w626:T4, "Tree Out"=w620:refnum<vi>)  [unwired: 3 in, 3 out]
            n255 = property class="Tree"(reference=w620, "Visible"=FALSE) -> (reference out=w625:refnum<vi>)  [unwired: 1 in, 1 out]
            n256 = for {
              tunnel: w626 -> [w665] mode=indexing
              tunnel: w630 -> [w650]
              shift-right: [w647] -> w622
              shift-left: w625 -> [w657]
              tunnel: [w646] -> w623 mode=indexing
              tunnel: w616 -> [w644]
              tunnel: w615 -> [w639]
              i -> [w649]
              w655 = ""
              n257 = Unbundle By Name(w665) -> ("StepNo&Category"=w645:string, "Tags"=w651:string[])
              n258 = Add(x=w650, y=w649) -> (x+y=w648:i32)
              n259 = case shown="\"GroupingbyStep\", Default" w644 {
                tunnel: [w666 w685] -> w641
                tunnel: w645 -> [w669 w678]
                tunnel: [w666 w679] -> w637
                tunnel: ["" ("StepNo&Category") w678] -> w636
                frame "GroupingbyCategory" {
                  n260 = case shown="\"Protected\"" w669 {
                    selector: w669 -> [w675 w677]
                    tunnel: [w670 w677] -> w667
                    frame Default {
                      n261 = String Subset(string=w675, length (rest)=3 ("length (rest)")) -> (substring=w671:string)  [unwired: 1 in]
                      n262 = Equal?(x="Seq", y=w671) -> (x = y?=w673:bool)
                      n263 = Select(t="Cal", s=w673, f=w671) -> (s? t:f=w670:string)
                    }
                    frame "Protected" {
                    }
                  }
                  n264 = call "CRYGet Category Name with MultiLang.vi"("Category"=w667) -> ("Name"=w666:string)  [unwired: 10 in]
                }
                frame "GroupingbyStep", Default {
                  n265 = global read "CRYCurve Library Global.vi" "ProtectDataStepNo"() -> (w684:i32)
                  n266 = Decimal String To Number(string=w678) -> (number=w680:i32)  [unwired: 2 in, 1 out]
                  n267 = Equal?(x=w684, y=w680) -> (x = y?=w683:bool)
                  n268 = case shown="False" w683 {
                    tunnel: [w686 w690] -> w685
                    tunnel: w680 -> [_ w691]
                    frame True {
                      n269 = call "CRYGet Category Name with MultiLang.vi"("Category"="Protected") -> ("Name"=w686:string)  [unwired: 10 in]
                    }
                    frame False {
                      n270 = call "CRYGet CurrentSteps By StepNo.vi"("Step Setup VI No"=w691) -> ("Step"=w702:T3)  [unwired: 8 in, 2 out]
                      n271 = Unbundle By Name(w702) -> ("Category"=w701:string, "StepName"=w695:string)
                      n272 = String Subset(string=w701, length (rest)=3 ("length (rest)")) -> (substring=w697:string)  [unwired: 1 in]
                      n273 = Equal?(x="Seq", y=w697) -> (x = y?=w692:bool)
                      n274 = Select(t="Calibration", s=w692, f=w695) -> (s? t:f=w693:string)
                      n275 = Select(t="Cal", s=w692, f=w697) -> (s? t:f=w689:string)
                      n276 = call "CRYGet Category Name with MultiLang.vi"("Category"=w689) -> ("Name"=w688:string)  [unwired: 10 in]
                      n277 = Concatenate Strings(w688, " - ", w693) -> (w690:string)
                    }
                  }
                  n278 = call "CRYGet Tree Number by StepNo.vi"("sOption"="ActualNumber", "Step Setup VI No"=w680) -> ("Number in Tree"=w682:i32)  [unwired: 8 in, 1 out]
                  n279 = Number To Decimal String(number=w682) -> (decimal integer string=w679:string)  [unwired: 1 in]
                }
              }
              n280 = call "CRYMake Name.vi"("sOption 2"="byCategory" ("sOption"), "Type"=w639, "sOption"="New", "sAction"="Group", "Name In"=w641) -> ("Name Out"=w640:string)  [unwired: 5 in, 1 out]
              n281 = Build Array(w655, w655, w641, w637, "Cat_Group" ("element"), w636) -> (w662:string[])
              n282 = invoke class="Tree" method="Edit Tree Items.Add Item"(reference=w657, "Parent Tag"="", "Child Position"=w648, "Left Cell"=w640, "Child Text"=w662, "Child Tag"=w640) -> (reference out=w664:refnum<vi>, error out=w653:errorcluster, "Edit Tree Items:Add Item"=w646:string)  [unwired: 3 in, 6 out]
              n283 = property class="Tree"(reference=w664, error in=w653, "Active Item Tag"=w646, "Glyph"=10 ("Active Item:Symbol Index"), "ActiveColNum"=0 ("Active Cell:Active Column Number"), "CellFontBold"=TRUE ("Active Cell:Cell Font:Bold"), "CellFontColor"=u32 16777228) -> (reference out=w654:refnum<vi>, error out=w652:errorcluster)
              n284 = for {
                tunnel: w652 -> [w707]
                tunnel: w646 -> [w706]
                shift-right: [w705] -> w647
                shift-left: w654 -> [w708]
                tunnel: w651 -> [w704] mode=indexing
                i -> [w703]
                n285 = invoke class="Tree" method="Edit Tree Items.Move Item"(reference=w708, error in=w707, "tag"=w704, "New Parent"=w706, "New Position"=w703) -> (reference out=w705:refnum<vi>)  [unwired: 2 in, 6 out]
              }
            }
            n286 = call "CRYGroup Manipulate Sub.vi"("sAction"="MakeGroupName", "sData"=w623, "Tree in"=w622) -> ("Tree Out"=w619:refnum<vi>, "sData Out"=w617:string[])  [unwired: 4 in, 3 out]
            n287 = for {
              shift-right: [w634] -> w618
              shift-left: w619 -> [w635]
              tunnel: w617 -> [w633] mode=indexing
              n288 = invoke class="Tree" method="Open/Close.Item"(reference=w635, "tag"=w633, "Open"=FALSE ("Open?")) -> (reference out=w634:refnum<vi>)  [unwired: 2 in, 4 out]
            }
            n289 = property class="Tree"(reference=w618, "Visible"=TRUE) -> ()  [unwired: 1 in, 2 out]
          }
        }
      }
    }
    frame "GroupingOff" {
      w713 = enum16{"Curves", "Values", "Results", "WFM"}[] [enum."Curves", enum."Values", enum."Results", enum."WFM"] items=["Curves", "Values", "Results", "WFM"]
      n290 = global read "CRYCurve Library Global.vi" "CurveLib Info"() -> (w712:T2)
      n291 = Unbundle By Name(w712) -> ("GroupingState"=w711:string)
      n292 = for {
        tunnel: w713 -> [w714] mode=indexing
        tunnel: w710 -> [w720]
        tunnel: w711 -> [w717]
        n293 = call "CRYTree Global Manipulate.vi"("sAction"="Get", "Type In"=w714) -> ("Tree/Curve Tree"=w730:refnum<vi>)  [unwired: 6 in, 3 out]
        n294 = Build Array("") -> (w740:string[])
        n295 = call "CRYTree Manipulate Sub.vi"("sAction"="GetTags", "sData"=w740, "sOption"="Childs", "Tree in"=w730) -> ("sData Out"=w737:string[], "Tree Out"=w733:refnum<vi>)  [unwired: 3 in, 3 out]
        n296 = for {
          tunnel: w737 -> [w763] mode=indexing
          tunnel: w733 -> [w768]
          shift-right: [w764] -> w726
          shift-left: string[] [] ("sData Out") -> [w765]
          # "Get Category Group"
          n297 = Build Array(w763) -> (w767:string[])
          n298 = call "CRYTree Manipulate Sub.vi"("sAction"="CheckGroup", "sData"=w767, "sOption"="byTag", "Tree in"=w768) -> ("bCategory"=w766:bool)  [unwired: 3 in, 4 out]
          n299 = case shown="True" w766 {
            tunnel: w765 -> [w771 w774]
            tunnel: [w771 w773] -> w764
            tunnel: w763 -> [_ w772]
            frame False {
            }
            frame True {
              n300 = Insert Into Array(array=w774, new element=w772) -> (w773:string[])  [unwired: 1 in]
            }
          }
        }
        n301 = call "CRYTree Manuplate.vi"("sAction"="FindInsertLoc", "sOption"="Grouping" ("sData"), "Tree in"=w730) -> ("nData Out"=w729:i32[])  [unwired: 5 in, 3 out]
        n302 = Index Array(array=w729) -> (element=w728:i32)  [unwired: 1 in]
        n303 = call "CRYTree Manipulate Sub.vi"("sAction"="GetTags", "sData"=w726, "sOption"="Childs", "Tree in"=w733) -> ("sData Out"=w716:string[], "Tree Out"=w719:refnum<vi>)  [unwired: 3 in, 3 out]
        n304 = case shown="\"Grouping by Category\"" w717 {
          tunnel: w719 -> [w743 w749]
          tunnel: [w743 w748] -> w718
          tunnel: w716 -> [w744 w747]
          tunnel: [w744 w746] -> w715
          tunnel: w714 -> [_ w745]
          frame "Grouping by Step", Default {
          }
          frame "Grouping by Category" {
            n305 = call "CRYGroup Manipulate Sub.vi"("Type"=w745, "sAction"="SortbyStepOrder", "sData"=w747, "Tree in"=w749) -> ("Tree Out"=w748:refnum<vi>, "sData Out"=w746:string[])  [unwired: 3 in, 3 out]
          }
        }
        n306 = property class="Tree"(reference=w718, "Visible"=FALSE) -> (reference out=w724:refnum<vi>)  [unwired: 1 in, 1 out]
        n307 = for {
          tunnel: w715 -> [w760] mode=indexing
          tunnel: w728 -> [w759]
          shift-right: [w756] -> w727
          shift-left: w724 -> [w762]
          i -> [w758]
          n308 = Add(x=w759, y=w758) -> (x+y=w757:i32)
          n309 = invoke class="Tree" method="Edit Tree Items.Move Item"(reference=w762, "tag"=w760, "New Parent"="", "New Position"=w757) -> (reference out=w756:refnum<vi>)  [unwired: 3 in, 6 out]
        }
        n310 = for {
          tunnel: w726 -> [w754] mode=indexing
          shift-right: [w753] -> w722
          shift-left: w727 -> [w755]
          n311 = invoke class="Tree" method="Edit Tree Items.Delete"(reference=w755, "tag"=w754) -> (reference out=w753:refnum<vi>)  [unwired: 3 in, 4 out]
        }
        n312 = property class="Tree"(reference=w722, "Value"=string[] []) -> (reference out=w721:refnum<vi>)  [unwired: 1 in, 1 out]
        n313 = case shown="\"Invisible\"" w720 {
          tunnel: w721 -> [_ w751]
          frame "Invisible" {
          }
          frame Default {
            n314 = property class="Tree"(reference=w751, "Visible"=TRUE) -> ()  [unwired: 1 in, 2 out]
          }
        }
      }
    }
    frame "ExistGroup" {
      # "CRYInsert Data to Listbox.vi"
      n315 = Index Array(array=w790) -> (element=w777:i32)  [unwired: 1 in]
      n316 = global read "CRYCurve Library Global.vi" "CurveLib Info"() -> (w782:T2)
      n317 = Unbundle By Name(w782) -> ("GroupingState"=w781:string)
      n318 = Build Array("") -> (w785:string[])
      n319 = call "CRYGet Group Category.vi"("sOption"="StepNo", "nData"=w777) -> ("sCategory"=w778:string)  [unwired: 9 in]
      n320 = call "CRYTree Manipulate Sub.vi"("sAction"="GetTags", "sData"=w785, "sOption"="Childs", "Tree in"=w791) -> ("sData Out"=w788:string[], "Tree Out"=w787:refnum<vi>)  [unwired: 3 in, 3 out]
      n321 = case shown="\"Grouping by Step\"" w781 {
        tunnel: w787 -> [w795 w812 _]
        tunnel: w777 -> [w796 _ _]
        tunnel: w788 -> [w794 w813 _]
        tunnel: [w793 w811 TRUE] -> w780
        tunnel: [w792 w810 "" ("sOption")] -> w779
        tunnel: w778 -> [_ w809 _]
        frame "Grouping by Step" {
          n322 = for {
            tunnel: w794 -> [w797] mode=indexing
            tunnel: w796 -> [w801]
            tunnel: w795 -> [w805]
            tunnel: [w798] -> w793
            tunnel: [w797] -> w792
            stop <- w798 stop-if-true
            n323 = Build Array(w797) -> (w806:string[])
            n324 = property class="Tree"(reference=w805, "Active Item Tag"=w797, "ActiveColNum"=6 ("Active Cell:Active Column Number")) -> ("Cell String"=w803:string)  [unwired: 1 in, 2 out]
            n325 = call "CRYTree Manipulate Sub.vi"("sAction"="CheckGroup", "sData"=w806, "sOption"="byTag", "Tree in"=w805) -> ("bCategory"=w799:bool)  [unwired: 3 in, 4 out]
            n326 = Decimal String To Number(string=w803) -> (number=w802:i32)  [unwired: 2 in, 1 out]
            n327 = Equal?(x=w802, y=w801) -> (x = y?=w800:bool)
            n328 = And(x=w799, y=w800) -> (x .and. y?=w798:bool)
          }
        }
        frame "Grouping by Category" {
          n329 = for {
            tunnel: w813 -> [w814] mode=indexing
            tunnel: w809 -> [w820]
            tunnel: w812 -> [w818]
            tunnel: [w815] -> w811
            tunnel: [w814] -> w810
            stop <- w815 stop-if-true
            n330 = Build Array(w814) -> (w822:string[])
            n331 = property class="Tree"(reference=w818, "Active Item Tag"=w814, "ActiveColNum"=4 ("Active Cell:Active Column Number")) -> ("Cell String"=w817:string)  [unwired: 1 in, 2 out]
            n332 = call "CRYTree Manipulate Sub.vi"("sAction"="CheckGroup", "sData"=w822, "sOption"="byTag", "Tree in"=w818) -> ("bCategory"=w816:bool)  [unwired: 3 in, 4 out]
            n333 = Equal?(x=w817, y=w820) -> (x = y?=w821:bool)
            n334 = And(x=w816, y=w821) -> (x .and. y?=w815:bool)
          }
        }
        frame "Grouping Off", Default {
        }
      }
      n335 = Build Array(w779) -> (w789:string[])
      n336 = local write "bData out"(w780) -> ()
      n337 = local write "sData Out"(w789) -> ()
    }
    frame "GroupRename" {
      w827 = enum16{"Curves", "Values", "Results", "WFM"}[] [enum."Curves", enum."Values", enum."Results", enum."WFM"] items=["Curves", "Values", "Results", "WFM"]
      # "StepName Change in Project Editor"
      n338 = Index Array(array=w837) -> (element=w836:i32)  [unwired: 1 in]
      n339 = call "CRYTree Global Manipulate.vi"("sAction"="Get", "sOption"="All") -> ("WFM Tree"=w829:refnum<vi>, "Results Tree"=w830:refnum<vi>, "Values Tree"=w831:refnum<vi>, "Tree/Curve Tree"=w832:refnum<vi>)  [unwired: 6 in]
      n340 = Build Array(w832, w831, w830, w829) -> (w828:refnum<vi>[])
      n341 = for {
        tunnel: w836 -> [w840]
        tunnel: w828 -> [w839] mode=indexing
        tunnel: w827 -> [w838] mode=indexing
        n342 = global read "CRYCurve Library Global.vi" "CurveLib Info"() -> (w842:T2)
        n343 = Unbundle By Name(w842) -> ("GroupingState"=w841:string)
        n344 = Build Array("") -> (w845:string[])
        n345 = call "CRYTree Manipulate Sub.vi"("sAction"="GetTags", "sData"=w845, "sOption"="Childs", "Tree in"=w839) -> ("sData Out"=w848:string[], "Tree Out"=w847:refnum<vi>)  [unwired: 3 in, 3 out]
        n346 = case shown="\"Grouping by Step\"" w841 {
          tunnel: w847 -> [w850 _]
          tunnel: w840 -> [w853 _]
          tunnel: w848 -> [w854 _]
          tunnel: w838 -> [w849 _]
          frame "Grouping by Step" {
            n347 = for {
              tunnel: w854 -> [w890] mode=indexing
              tunnel: w853 -> [w894]
              tunnel: w850 -> [w898]
              tunnel: [w891] -> w852
              tunnel: [w890] -> w851
              stop <- w891 stop-if-true
              n348 = Build Array(w890) -> (w899:string[])
              n349 = property class="Tree"(reference=w898, "Active Item Tag"=w890, "ActiveColNum"=6 ("Active Cell:Active Column Number")) -> ("Cell String"=w896:string)  [unwired: 1 in, 2 out]
              n350 = call "CRYTree Manipulate Sub.vi"("sAction"="CheckGroup", "sData"=w899, "sOption"="byTag", "Tree in"=w898) -> ("bCategory"=w892:bool)  [unwired: 3 in, 4 out]
              n351 = Decimal String To Number(string=w896) -> (number=w895:i32)  [unwired: 2 in, 1 out]
              n352 = Equal?(x=w895, y=w894) -> (x = y?=w893:bool)
              n353 = And(x=w892, y=w893) -> (x .and. y?=w891:bool)
            }
            n354 = case shown="True" w852 {
              tunnel: w853 -> [w878 _]
              tunnel: w851 -> [w855 _]
              tunnel: w850 -> [w869 _]
              tunnel: w849 -> [w856 _]
              frame True {
                n355 = call "CRYGet CurrentSteps By StepNo.vi"("Step Setup VI No"=w878) -> ("Step"=w889:T3)  [unwired: 8 in, 2 out]
                n356 = Unbundle By Name(w889) -> ("Category"=w888:string, "StepName"=w882:string)
                n357 = String Subset(string=w888, length (rest)=3 ("length (rest)")) -> (substring=w884:string)  [unwired: 1 in]
                n358 = Equal?(x="Seq", y=w884) -> (x = y?=w879:bool)
                n359 = Select(t="Calibration", s=w879, f=w882) -> (s? t:f=w880:string)
                n360 = Select(t="Cal", s=w879, f=w884) -> (s? t:f=w877:string)
                n361 = call "CRYGet Category Name with MultiLang.vi"("Category"=w877) -> ("Name"=w876:string)  [unwired: 10 in]
                n362 = Concatenate Strings(w876, " - ", w880) -> (w868:string)
                n363 = call "CRYMake Name.vi"("sOption 2"="byCategory" ("sOption"), "Type"=w856, "sOption"="New", "sAction"="Group", "Name In"=w868) -> ("Name Out"=w860:string)  [unwired: 5 in, 1 out]
                n364 = Reverse String(1:w855) -> (0:w866:string)
                n365 = Match Pattern(string=w866, regular expression="\\(" ("search string/char (-)")) -> (before substring=w864:string, match substring=w863:string)  [unwired: 1 in, 2 out]
                n366 = Concatenate Strings(w864, w863) -> (w861:string)
                n367 = Reverse String(1:w861) -> (0:w862:string)
                n368 = call <vilib>:"Trim Whitespace.vi"("string"=w862) -> ("trimmed string"=w858:string)  [unwired: 1 in]
                n369 = call <vilib>:"Space Constant.vi"() -> ("String"=w859:string)
                n370 = Concatenate Strings(w860, w859, w858) -> (w857:string)
                n371 = property class="Tree"(reference=w869, "Active Item Tag"=w855, "ActiveColNum"=0 ("Active Cell:Active Column Number"), "Cell String"=w857, "ActiveColNum"=3 ("Active Cell:Active Column Number"), "Cell String"=w868) -> (reference out=w867:refnum<vi>, "Active Item Tag"=w871:string)  [unwired: 1 in, 1 out]
                n372 = invoke class="Tree" method="Edit Tree Items.Set Tag"(reference=w867, "tag"=w871, "new tag"=w857) -> ()  [unwired: 2 in, 5 out]
              }
              frame False {
              }
            }
          }
          frame "Grouping Off", Default {
          }
        }
      }
    }
    frame "MakeGroup" {
      w932 = ""
      # "CRYInsert Data to Listbox.vi"
      n373 = Index Array(array=w916) -> (element=w905:i32)  [unwired: 1 in]
      n374 = global read "CRYCurve Library Global.vi" "CurveLib Info"() -> (w936:T2)
      n375 = Unbundle By Name(w936) -> ("GroupingState"=w914:string)
      n376 = call "CRYGet Tree Number by StepNo.vi"("sOption"="ActualNumber", "Step Setup VI No"=w905) -> ("Number in Tree"=w903:i32)  [unwired: 8 in, 1 out]
      n377 = case shown="\"Grouping by Category\"" w914 {
        tunnel: [w938 w955] -> w907
        tunnel: w905 -> [_ w950]
        tunnel: [w938 w952] -> w915
        tunnel: w903 -> [w941 w951]
        tunnel: ["" w949] -> w904
        frame "Grouping by Category" {
          n378 = call "CRYGet Group Category.vi"("sOption"="VisibleIndex", "nData"=w941) -> ("sCategory"=w942:string)  [unwired: 9 in]
          n379 = case shown="Default" w942 {
            selector: w942 -> [w943 w948]
            tunnel: [w944 w948] -> w938
            frame Default {
              n380 = Equal?(x="Seq", y=w943) -> (x = y?=w946:bool)
              n381 = Select(t="Cal", s=w946, f=w943) -> (s? t:f=w944:string)
            }
            frame "Protected", "保护" {
            }
          }
        }
        frame "Grouping by Step", Default {
          n382 = global read "CRYCurve Library Global.vi" "ProtectDataStepNo"() -> (w954:i32)
          n383 = Equal?(x=w954, y=w950) -> (x = y?=w953:bool)
          n384 = case shown="False" w953 {
            tunnel: [w956 w968] -> w955
            tunnel: w950 -> [_ w960]
            frame True {
              n385 = call "CRYGet Category Name with MultiLang.vi"("Category"="Protected") -> ("Name"=w956:string)  [unwired: 10 in]
            }
            frame False {
              n386 = call "CRYGet CurrentSteps By StepNo.vi"("Step Setup VI No"=w960) -> ("Step"=w972:T3)  [unwired: 8 in, 2 out]
              n387 = Unbundle By Name(w972) -> ("Category"=w971:string, "StepName"=w964:string)
              n388 = String Subset(string=w971, length (rest)=3 ("length (rest)")) -> (substring=w966:string)  [unwired: 1 in]
              n389 = Equal?(x="Seq", y=w966) -> (x = y?=w961:bool)
              n390 = Select(t="Calibration", s=w961, f=w964) -> (s? t:f=w962:string)
              n391 = Select(t="Cal", s=w961, f=w966) -> (s? t:f=w959:string)
              n392 = call "CRYGet Category Name with MultiLang.vi"("Category"=w959) -> ("Name"=w958:string)  [unwired: 10 in]
              n393 = Concatenate Strings(w958, " - ", w962) -> (w968:string)
            }
          }
          n394 = Number To Decimal String(number=w951) -> (decimal integer string=w952:string)  [unwired: 1 in]
          n395 = Number To Decimal String(number=w950) -> (decimal integer string=w949:string)  [unwired: 1 in]
        }
      }
      n396 = call "CRYMake Name.vi"("sOption 2"="byCategory" ("sOption"), "Type"=w909, "sOption"="New", "sAction"="Group", "Name In"=w907) -> ("Name Out"=w908:string)  [unwired: 5 in, 1 out]
      n397 = Build Array(w903) -> (w922:i32[])
      n398 = Build Array(w932, w932, w907, w915, "Cat_Group" ("element"), w904) -> (w934:string[])
      n399 = call "CRYTree Manuplate.vi"("sAction"="FindInsertLoc", "nData"=w922, "sOption"="StepDataGroup" ("sData"), "Tree in"=w937) -> ("nData Out"=w924:i32[], "Tree Out"=w925:refnum<vi>)  [unwired: 4 in, 2 out]
      n400 = Index Array(array=w924) -> (element=w923:i32)  [unwired: 1 in]
      n401 = invoke class="Tree" method="Edit Tree Items.Add Item"(reference=w925, "Parent Tag"="", "Child Position"=w923, "Left Cell"=w908, "Child Text"=w934, "Child Tag"=w908) -> (reference out=w928:refnum<vi>, "Edit Tree Items:Add Item"=w918:string)  [unwired: 3 in, 7 out]
      n402 = property class="Tree"(reference=w928, "Active Item Tag"=w918, "Glyph"=10 ("Active Item:Symbol Index"), "ActiveColNum"=0 ("Active Cell:Active Column Number"), "CellFontBold"=TRUE ("Active Cell:Cell Font:Bold"), "CellFontColor"=u32 16777228) -> (reference out=w919:refnum<vi>)  [unwired: 1 in, 1 out]
      n403 = Build Array(w918) -> (w920:string[])
      n404 = call "CRYGroup Manipulate Sub.vi"("sAction"="MakeGroupName", "sData"=w920, "Tree in"=w919) -> ("sData Out"=w917:string[])  [unwired: 4 in, 4 out]
      n405 = local write "sData Out"(w917) -> ()
    }
  }
  n406 = case shown="\"SequenceInsert\", \"StepInsert\", \"StepMoveDown\", \"StepMoveUp\", \"StepRemove\"" w2 {
    frame Default {
    }
    frame "SequenceInsert", "StepInsert", "StepMoveDown", "StepMoveUp", "StepRemove" {
      # "If the case is StepMoveDown or StepMoveUp,\nit is processde in \nCRYProject\\SubVI\\CRYUpdate TS Structure.vi"
      n407 = global read "CRYCurve Library Global.vi" "CurveLib Info"() -> (w974:T2)
      n408 = Unbundle By Name(w974) -> ("GroupingState"=w973:string)
      n409 = case shown="\"Grouping by Step\"" w973 {
        frame Default {
        }
        frame "Grouping by Step" {
          n410 = call "CRYGroup Manipulate Sub.vi"("sAction"="ChangeTreeNum") -> ()  [unwired: 6 in, 5 out]
        }
      }
    }
  }
  "Tree Out" <- "Tree in"
